vi "Edit Message.vi"(8 "error in (no error)":errorcluster, 10 "Flex Msg in":refnum<class "Flex Msg.lvclass">, 11 "Sequence Element in":T1) -> (0 "error out":errorcluster, 3 "Sequence Element out":T1)   [LabVIEW 2020, in "Sequencer.lvlib"]
doc: "Edit the private data of a Flex Msg and setup data override."
uses:
  Sequencer.lvlib
  Controls/Ctl_SequenceElement.ctl
  Controls/Ctl_SequenceControlElement.ctl
  PPL/HDH.Actor Framework.Core.Msg.lvlibp/Flex Msg/Controls/Ctl_Control Element.ctl
  PPL/HDH.Actor Framework.Core.Msg.lvlibp/Flex Msg/Flex Msg.lvclass
  PPL/HDH.Actor Framework.Core.Msg.lvlibp/Flex Msg/Data Access Handlers/Get Refnum/Get Refnum.lvclass
  C:/Current projects/WS/PPL/HDH.Actor Framework.Core.Msg.lvlibp/Flex Msg/Data Access Handlers/Data Access Handler/Data Access Handler.lvclass
  PPL/HDH.Actor Framework.Core.Msg.lvlibp
panel:
  in  "Looped?":bool
  in  "Control Data Override name":string
  in  "Controls":i32(listbox)
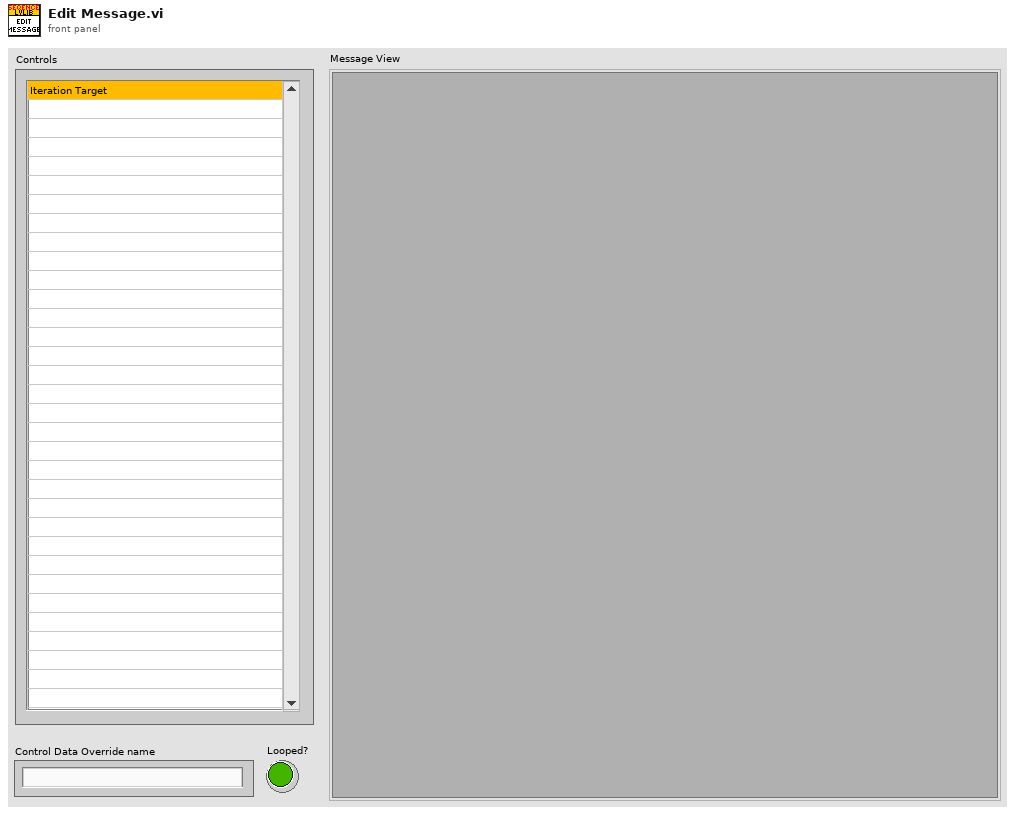
[diagram p1: front panel]
types:
  T1 = typedef "Sequencer.lvlib/Ctl_SequenceElement.ctl" = cluster{"Message Base Name":string, "Message Path":path, "Supports Data Access?":bool, "List Symbol":i32, "Sequence Control Element Array":T2[]}
  T2 = typedef "Sequencer.lvlib/Ctl_SequenceControlElement.ctl" = cluster{"Data Override name":string, "Looped Override?":bool, "Control element":T3, "List Symbol":i32}
  T3 = typedef "HDH.Actor Framework.Core.Msg.lvlibp/Ctl_Control Element.ctl" = cluster{"Index":i32, "Label":string, "Value":variant}
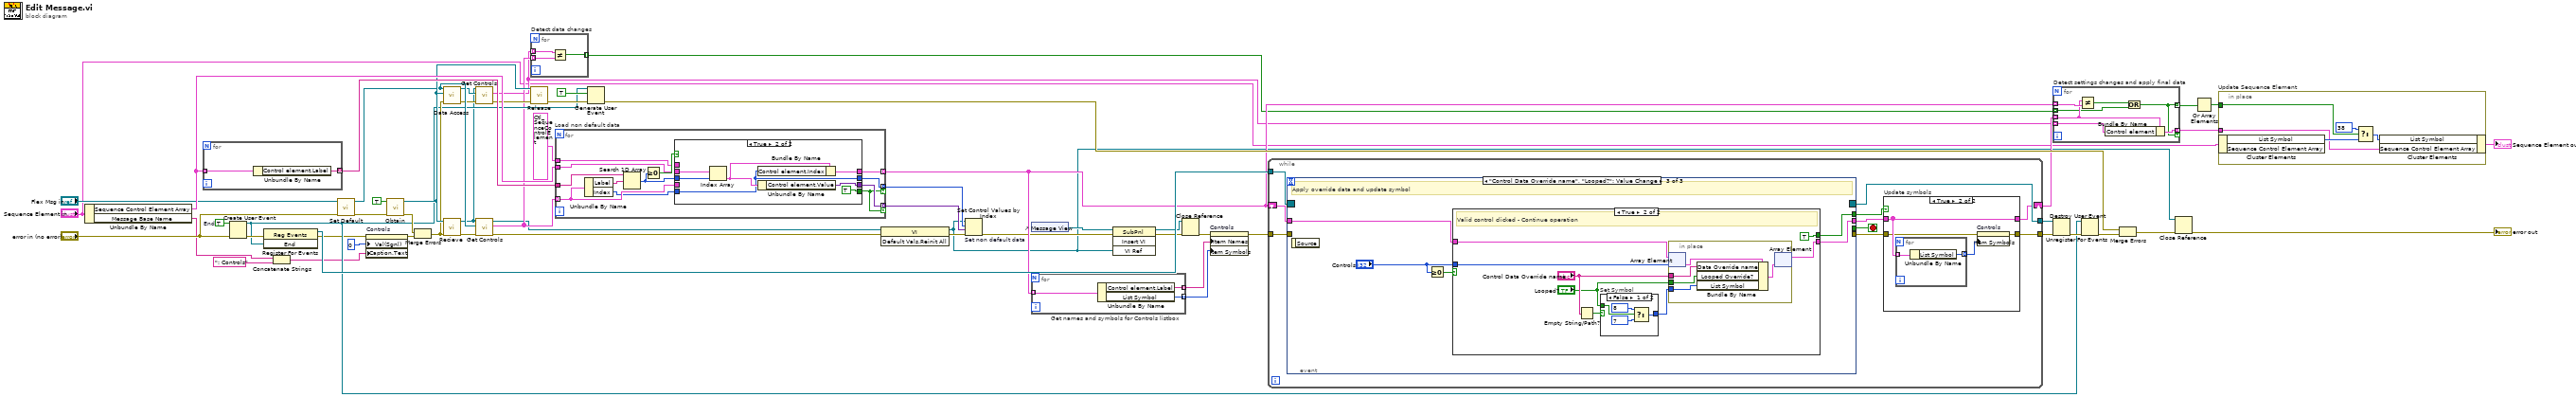
[diagram p0: block diagram]
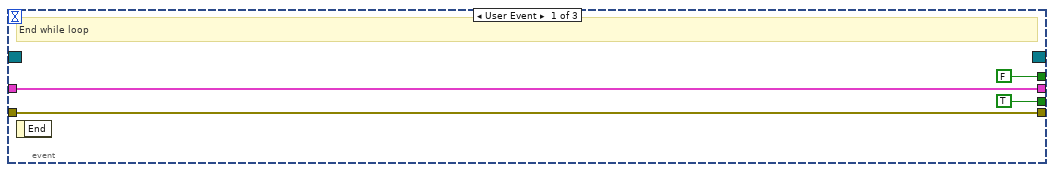
[diagram p3: hidden frame]
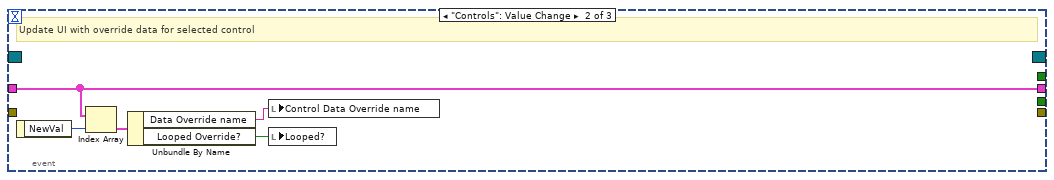
[diagram p4: hidden frame]
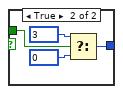
[diagram p6: hidden frame]
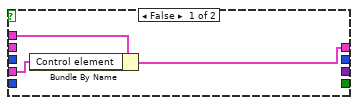
[diagram p7: hidden frame]
diagram:
  w44 = TRUE  # End
  n1 = Unbundle By Name("Sequence Element in") -> ("Sequence Control Element Array"=w54:T2[], "Message Base Name"=w12:string)
  n2 = for {
    tunnel: w54 -> [w61] mode=indexing
    tunnel: [w60] -> w56 mode=indexing
    n3 = Unbundle By Name(w61) -> ("Control element.Label"=w60:string)
  }
  n4 = Create User Event(user event datatype=w44, error in="error in (no error)") -> (user event=w35:refnum<user-event>, error out=w42:errorcluster)
  n5 = register-events(error in=w42, w35) -> (reference out=w38:refnum<event-registration>, error out=w28:errorcluster)  [unwired: 1 in]
  n6 = Concatenate Strings(w12, ": Controls" ("Caption.Text")) -> (w8:string)
  n7 = call-dynamic "Set Default.vi"("error in (no error)"="error in (no error)", "Flex Msg in"="Flex Msg in") -> ("error out"=w45:errorcluster, "Flex Msg out"=w46:refnum<class "Flex Msg.lvclass">)  [unwired: 8 in]
  n8 = property on="Controls" class="LstBox (strict)"(error in=w28, "Val(Sgnl)"=0 ("Value (Signaling)"), "Caption.Text"=w8) -> (error out=w27:errorcluster)  [unwired: 1 in, 1 out]
  n9 = call "Obtain.vi"("error in (no error)"=w45, "Await interaction?(F)"=TRUE) -> ("error out"=w58:errorcluster, "Get Refnum out"=w51:refnum<class "Get Refnum.lvclass">)  [unwired: 8 in]
  n10 = Merge Errors(w58, w27) -> (w41:errorcluster)
  n11 = call-dynamic "Data Access.vi"("error in (no error)"=w41, "Data Access Handler"=w51, "Flex Msg in"=w46) -> ("error out"=w26:errorcluster, "Flex Msg out"=w24:refnum<class "Flex Msg.lvclass">)  [unwired: 7 in]
  n12 = call "Recieve.vi"("error in (no error)"=w41, "Get Refnum in"=w51) -> ("error out"=w57:errorcluster, "VI Refnum"=w23:refnum<vi>)  [unwired: 7 in, 1 out]
  n13 = call "Get Controls.vi"("error in (no error)"=w26, "Flex Msg in"=w24, "VI Refnum in"=w23) -> ("error out"=w25:errorcluster, "Control Element Array"=w19:T3[])  [unwired: 6 in, 1 out]
  n14 = call "Get Controls.vi"("error in (no error)"=w57, "Flex Msg in"=w46, "VI Refnum in"=w23) -> ("error out"=w6:errorcluster, "Control Element Array"=w22:T3[], "VI Refnum out"=w7:refnum<vi>)  [unwired: 6 in]
  n15 = for "Detect data changes" {
    tunnel: w19 -> [w64] mode=indexing
    tunnel: w22 -> [w63] mode=indexing
    tunnel: [w62] -> w18 mode=indexing
    n16 = Not Equal?(x=w64, y=w63) -> (x != y?=w62:bool)
  }
  n17 = call "Release.vi"("error in (no error)"=w25, "Get Refnum in"=w51) -> ("error out"=w40:errorcluster)  [unwired: 9 in]
  n18 = for "Load non default data" {
    tunnel: w22 -> [w73] mode=indexing
    tunnel: w56 -> [w74]
    tunnel: T2 {"Data Override name"="", "Looped Override?"=FALSE, "Control element"={"Index"=0, "Label"="", "Value"=variant}, "List Symbol"=0} ("Sequence Control Element") -> [w68]
    tunnel: w54 -> [w71]
    tunnel: [w69] -> w20 mode=indexing
    tunnel: [w67] -> w53 mode=indexing if=w65
    tunnel: [w66] -> w52 mode=indexing if=w65
    n19 = Unbundle By Name(w73) -> ("Label"=w76:string, "Index"=w70:i32)
    n20 = Search 1D Array(1D array=w74, element=w76) -> (index of element=w72:i32)  [unwired: 1 in]
    n21 = Greater Or Equal To 0?(x=w72) -> (x >= 0?=w75:bool)
    n22 = case shown="True" w75 {
      tunnel: w71 -> [_ w86]
      tunnel: w73 -> [w77 _]
      tunnel: w72 -> [_ w85]
      tunnel: w70 -> [_ w81]
      tunnel: [w78 w84] -> w69
      tunnel: w68 -> [w79 _]
      tunnel: [_ w82] -> w67
      tunnel: [_ w81] -> w66
      tunnel: [_ TRUE] -> w65
      frame False {
        n23 = Bundle By Name(cluster=w79, "Control element"=w77) -> (w78:T2)
      }
      frame True {
        n24 = Index Array(array=w86, index=w85) -> (element=w83:T2)
        n25 = Bundle By Name(cluster=w83, "Control element.Index"=w81) -> (w84:T2)
        n26 = Unbundle By Name(w83) -> ("Control element.Value"=w82:variant)
      }
    }
  }
  n27 = Generate User Event(user event=w35, event data cluster=TRUE ("event data"), error in=w40) -> (error out=w33:errorcluster)  [unwired: 1 in, 1 out]
  n28 = invoke class="VI" method="Default Vals.Reinit All"(reference=w7, error in=w6) -> (reference out=w2:refnum<vi>, error out=w5:errorcluster)  [unwired: 1 in, 1 out]
  n29 = Set Control Values by Index "Set non default data"(0:w2, 1:w52, 2:w53, 3:w5) -> (11:w4:errorcluster)
  n30 = control-ref of="Message View"() -> (w50:refnum<vi>)
  n31 = for "Get names and symbols for Controls listbox" {
    tunnel: w20 -> [w89] mode=indexing
    tunnel: [w88] -> w49 mode=indexing
    tunnel: [w87] -> w48 mode=indexing
    n32 = Unbundle By Name(w89) -> ("Control element.Label"=w88:string, "List Symbol"=w87:i32)
  }
  n33 = invoke class="SubPnl" method="Insert VI"(reference=w50, error in=w4, "VI Ref"=w2) -> (reference out=w11:refnum<vi>, error out=w10:errorcluster)  [unwired: 1 in, 2 out]
  n34 = Close Reference(reference=w11, error in (no error)=w10) -> (error out=w1:errorcluster)
  n35 = property on="Controls" class="LstBox (strict)"(error in=w1, "Item Names"=w49, "Item Symbols"=w48) -> (error out=w34:errorcluster)  [unwired: 1 in, 1 out]
  n36 = while {
    tunnel: w38 -> [w99]
    tunnel: [w98] -> w37
    shift-right: [w93] -> w21
    shift-left: w20 -> [w95]
    tunnel: [w92] -> w31
    tunnel: w34 -> [w90]
    stop <- w97 stop-if-true
    n37 = event shown="[2] \"Control Data Override name\", \"Looped?\": Value Change" {
      selector: w99 -> [_ _ _]
      dyn-events: [_ _ _] -> w98
      timeout: _ -> [_ _ _]
      tunnel: [TRUE _ _] -> w97
      tunnel: [FALSE _ w117] -> w96
      tunnel: w95 -> [w109 w115 w121]
      tunnel: [w109 w115 w119] -> w94
      tunnel: [w108 _ _] -> w91
      tunnel: w90 -> [w108 _ _]
      event User Event {
        # "End while loop"
        n38 = event-data() -> ()  [unwired: 1 in, 1 out]
      }
      event "Controls": Value Change {
        # "Update UI with override data for selected control"
        n39 = event-data() -> ("NewVal"=w116:i32)  [unwired: 1 in]
        n40 = Index Array(array=w115, index=w116) -> (element=w114:T2)
        n41 = Unbundle By Name(w114) -> ("Data Override name"=w113:string, "Looped Override?"=w112:bool)
        n42 = local write "Control Data Override name"(w113) -> ()
        n43 = local write "Looped?"(w112) -> ()
      }
      event "Control Data Override name", "Looped?": Value Change {
        # "Apply override data and update symbol"
        n44 = event-data() -> ()  [unwired: 1 in, 1 out]
        n45 = Greater Or Equal To 0?(x="Controls") -> (x >= 0?=w120:bool)
        n46 = case shown="True" w120 {
          tunnel: w121 -> [w122 w130]
          tunnel: [w122 w125] -> w119
          tunnel: "Controls" -> [_ w124]
          tunnel: [_ TRUE] -> w117
          frame False {
            # "Invalid control clicked"
          }
          frame True {
            # "Valid control clicked - Continue operation"
            n47 = Empty String/Path?(string/path="Control Data Override name") -> (empty?=w128:bool)
            n48 = case "Set Symbol" shown="False" w128 {
              tunnel: "Looped?" -> [w134 w138]
              tunnel: [w131 w135] -> w126
              frame False {
                n49 = Select(t=8, s=w134, f=7) -> (s? t:f=w131:i32)
              }
              frame True {
                n50 = Select(t=3, s=w138, f=0) -> (s? t:f=w135:i32)
              }
            }
            n51 = in-place {
              in-place-border: "Control Data Override name" -> [w142]
              in-place-border: "Looped?" -> [w141]
              in-place-border: w126 -> [w139]
              n52 = in-place-array #1(w130, w124) -> (w143:T2)
              n53 = Bundle By Name(cluster=w143, "Data Override name"=w142, "Looped Override?"=w141, "List Symbol"=w139) -> (w140:T2)
              n54 = in-place-array #1(w140) -> (w125:T2[])  [unwired: 1 out]
            }
          }
        }
      }
    }
    n55 = case "Update symbols" shown="True" w96 {
      tunnel: w94 -> [w101 w104]
      tunnel: [w101 w104] -> w93
      tunnel: [w100 w102] -> w92
      tunnel: w91 -> [w100 w103]
      frame False {
      }
      frame True {
        n56 = for {
          tunnel: w104 -> [w107] mode=indexing
          tunnel: [w106] -> w105 mode=indexing
          n57 = Unbundle By Name(w107) -> ("List Symbol"=w106:i32)
        }
        n58 = property on="Controls" class="LstBox (strict)"(error in=w103, "Item Symbols"=w105) -> (error out=w102:errorcluster)  [unwired: 1 in, 1 out]
      }
    }
  }
  n59 = for "Detect settings changes and apply final data" {
    tunnel: w21 -> [w149] mode=indexing
    tunnel: w20 -> [w150] mode=indexing
    tunnel: w19 -> [w148] mode=indexing
    tunnel: [w147] -> w14 mode=indexing if=w144
    tunnel: w18 -> [w145] mode=indexing
    tunnel: [w144] -> w17 mode=indexing
    n60 = Not Equal?(x=w149, y=w150) -> (x != y?=w146:bool)
    n61 = Bundle By Name(cluster=w149, "Control element"=w148) -> (w147:T2)
    n62 = Or(x=w146, y=w145) -> (x .or. y?=w144:bool)
  }
  n63 = Unregister For Events(event registration refnum=w37, error in=w31) -> (error out=w36:errorcluster)
  n64 = Destroy User Event(user event=w35, error in=w36) -> (error out=w30:errorcluster)
  n65 = Merge Errors(w33, w30) -> (w32:errorcluster)
  n66 = Close Reference(reference=w2, error in (no error)=w32) -> (error out=→"error out":errorcluster)
  n67 = Or Array Elements(Boolean array=w17) -> (logical OR=w15:bool)
  n68 = in-place "Update Sequence Element" {
    in-place-border: w15 -> [w155]
    in-place-border: w14 -> [w151]
    n69 = in-place-cluster #2("Sequence Element in") -> ("List Symbol"=w154:i32)  [unwired: 1 out]
    n70 = Select(t=38, s=w155, f=w154) -> (s? t:f=w152:i32)
    n71 = in-place-cluster #2("List Symbol"=w152, "Sequence Control Element Array"=w151) -> (→"Sequence Element out":T1)
  }
